vi "Table Select 2.vi"() -> ()   [LabVIEW 2019]
uses:
  Ctrl/Table Save.ctl
  LLB/Commonly VI.lvlib
panel:
  out "S14 Table":string[][](array[string])
  out "S1 Table":string[][](array[string])
  out "EnfMeasureTable":cluster{"Table Control":string[][]}[](array[cluster])
  in  "Tab Control":enum32{"Page 1", "Page 2", "Page 3", "Page 4"}(tab)
  out "S4 Table":string[][](array[string])
  out "S3 Table":string[][](array[string])
  out "S2 Table":string[][](array[string])
  out "S5 Table":string[][](array[string])
  out "S6 Table":string[][](array[string])
  out "S7 Table":string[][](array[string])
  out "S8 Table":string[][](array[string])
  out "S9 Table":string[][](array[string])
  out "S10 Table":string[][](array[string])
  out "S11 Table":string[][](array[string])
  out "S12 Table":string[][](array[string])
  out "S13 Table":string[][](array[string])
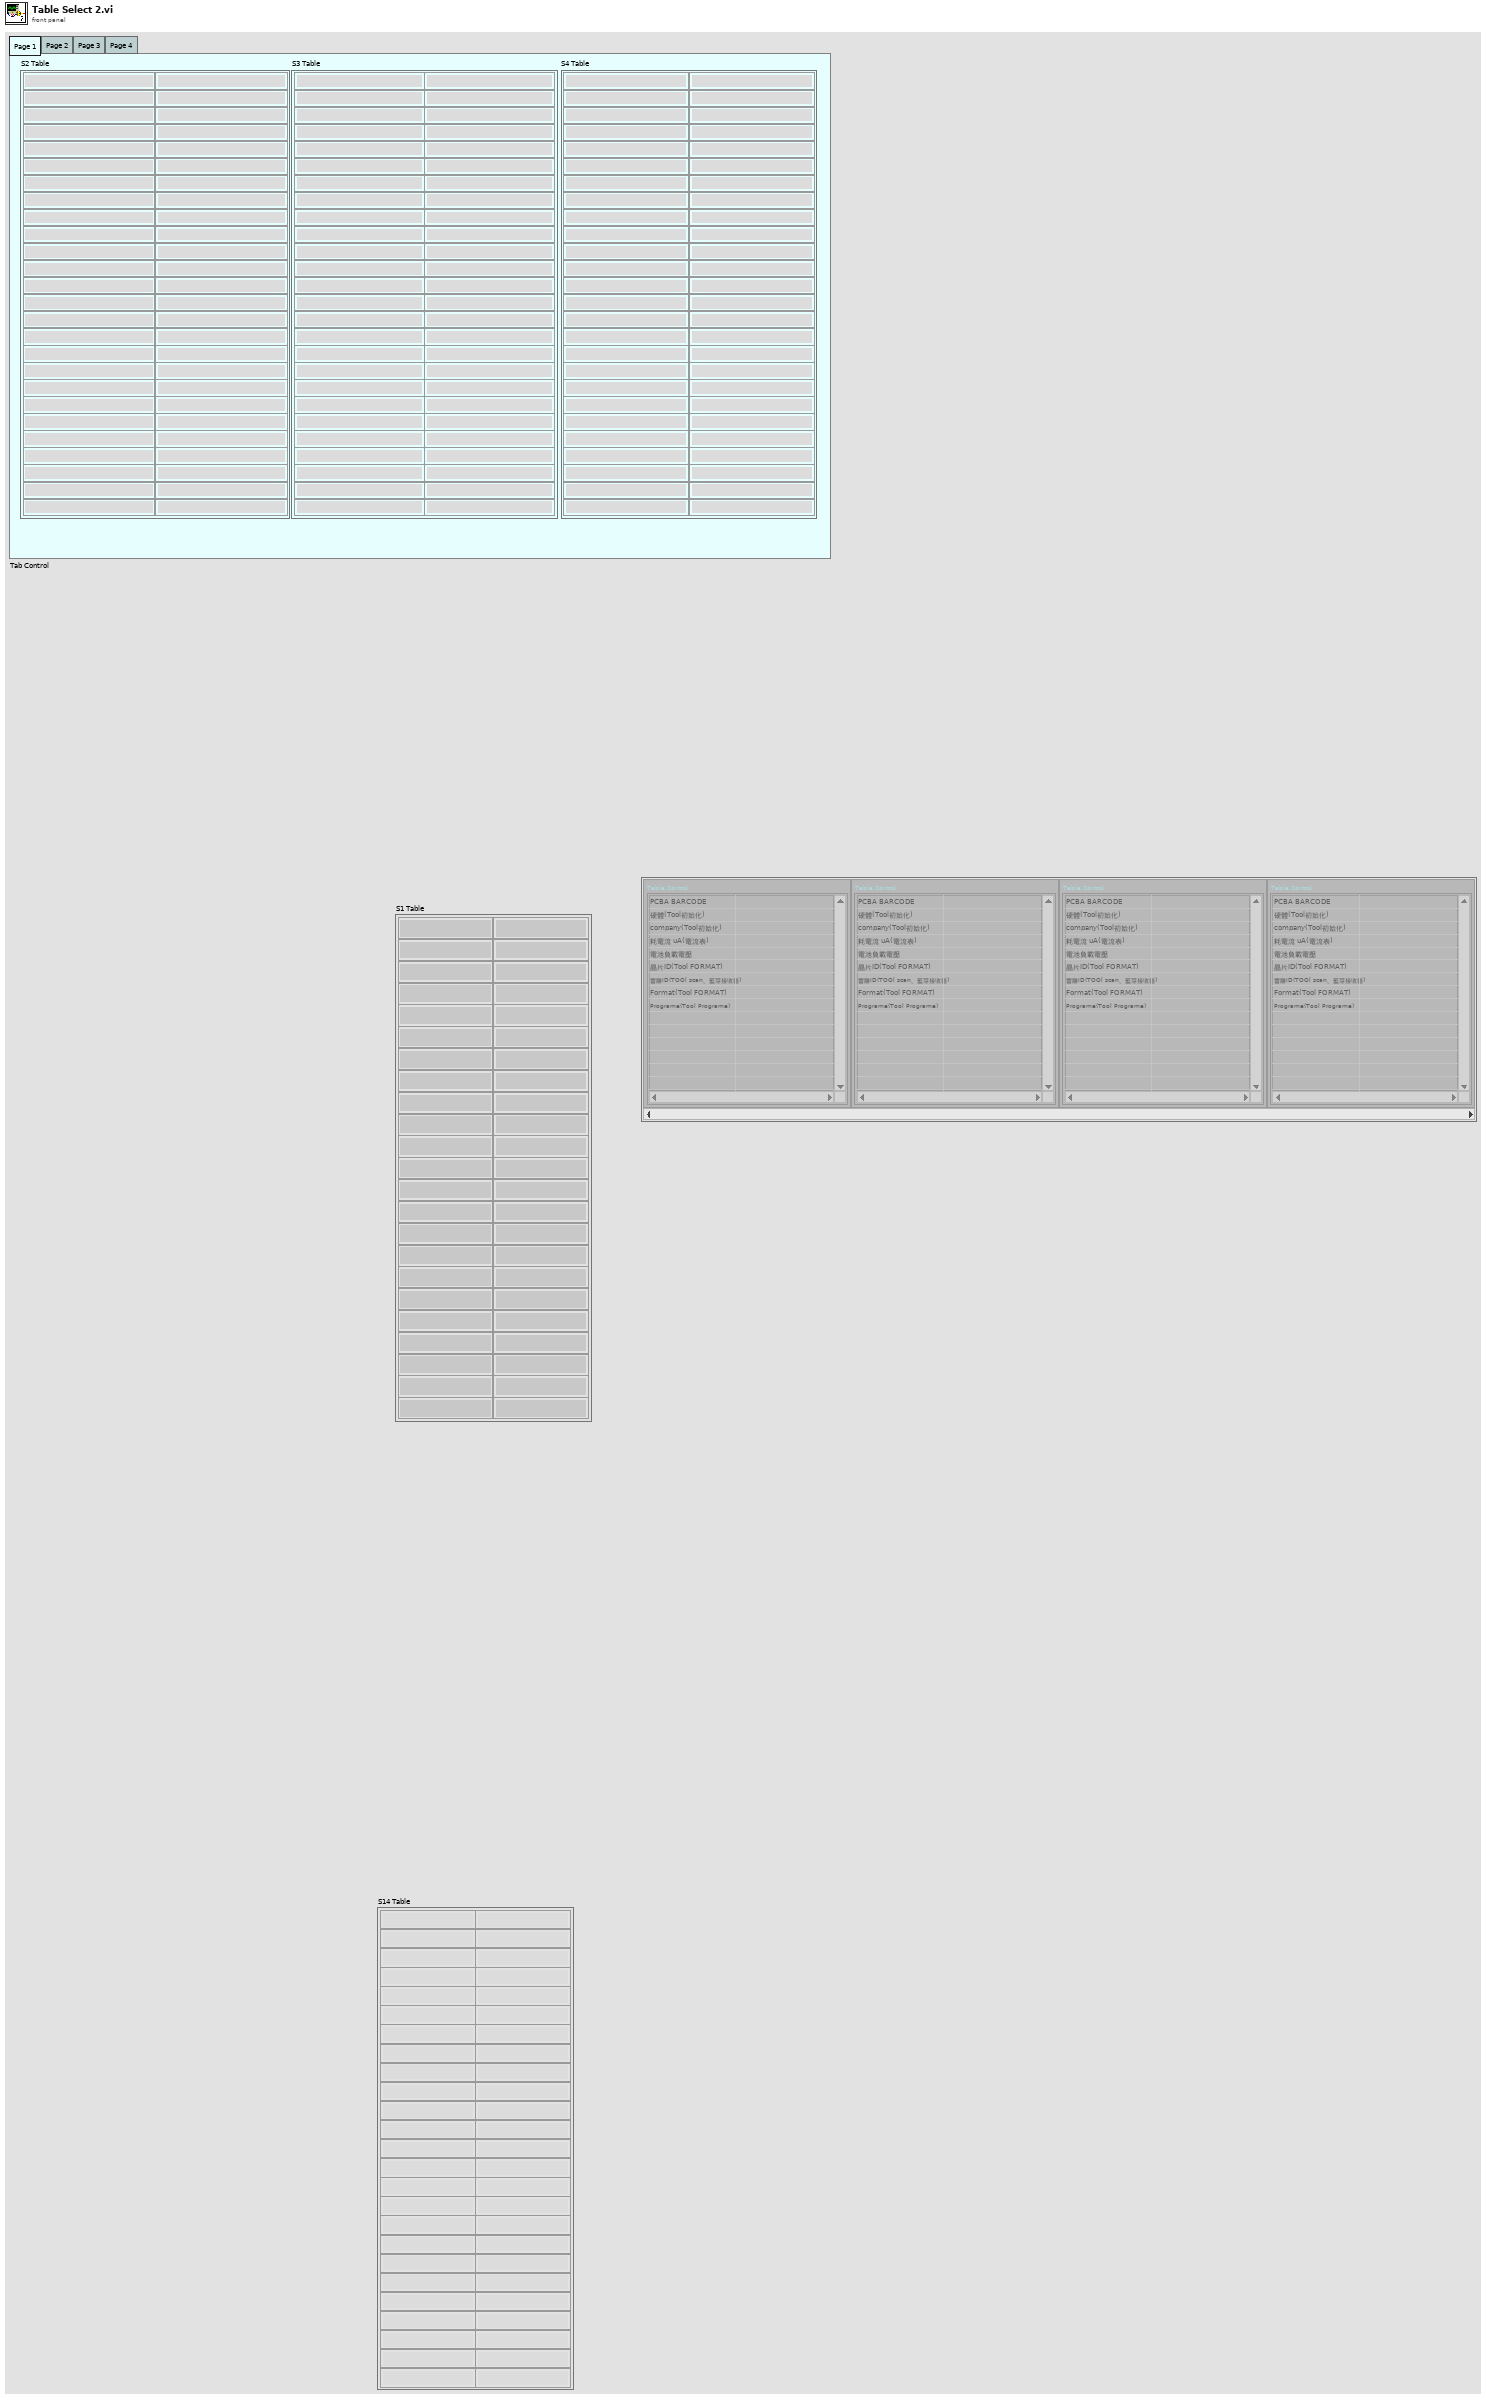
[diagram p1: front panel]
types:
  T1 = typedef "Table Save.ctl" = enum16{"initial", "Add", "Write", "Replace", "Delete", "REad", "RedTable", "Load"}
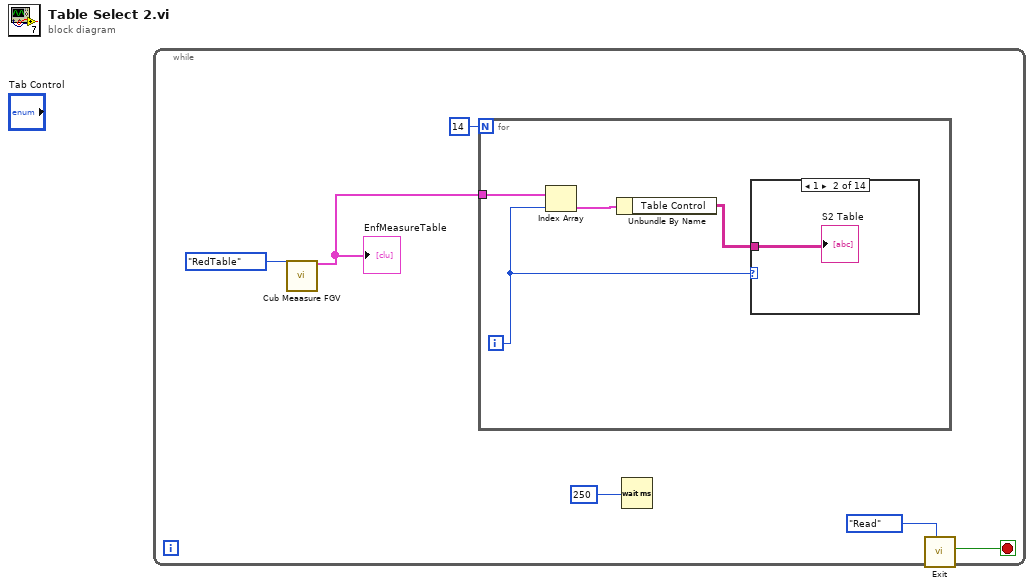
[diagram p0: block diagram]
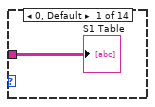
[diagram p2: hidden frame]
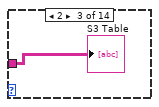
[diagram p3: hidden frame]
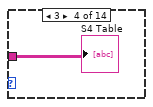
[diagram p4: hidden frame]
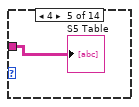
[diagram p5: hidden frame]
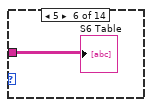
[diagram p6: hidden frame]
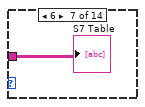
[diagram p7: hidden frame]
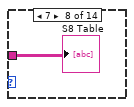
[diagram p8: hidden frame]
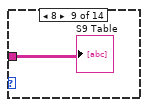
[diagram p9: hidden frame]
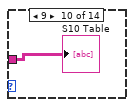
[diagram p10: hidden frame]
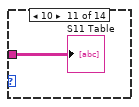
[diagram p11: hidden frame]
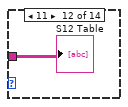
[diagram p12: hidden frame]
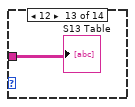
[diagram p13: hidden frame]
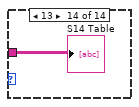
[diagram p14: hidden frame]
diagram:
  n1 = while {
    stop <- w2 stop-if-true
    n2 = call "Cub Meaasure FGV.vi"("Action"=Table_Save."RedTable" ("Enum")) -> ("Total Table"=w5:cluster{"Table Control":string[][]}[])  [unwired: 11 in, 7 out]
    "EnfMeasureTable" <- w5
    n3 = for {
      N: 14 -> [_]
      tunnel: w5 -> [w9]
      i -> [w8]
      n4 = Index Array(array=w9, index=w8) -> (element=w10:cluster{"Table Control":string[][]})
      n5 = Unbundle By Name(w10) -> ("Table Control"=w7:string[][])
      n6 = case shown="1" w8 {
        tunnel: w7 -> [w11 w12 w13 w14 w15 w16 w17 w18 w19 w20 w21 w22 w23 w24]
        frame 0, Default {
          "S1 Table" <- w11
        }
        frame 1 {
          "S2 Table" <- w12
        }
        frame 2 {
          "S3 Table" <- w13
        }
        frame 3 {
          "S4 Table" <- w14
        }
        frame 4 {
          "S5 Table" <- w15
        }
        frame 5 {
          "S6 Table" <- w16
        }
        frame 6 {
          "S7 Table" <- w17
        }
        frame 7 {
          "S8 Table" <- w18
        }
        frame 8 {
          "S9 Table" <- w19
        }
        frame 9 {
          "S10 Table" <- w20
        }
        frame 10 {
          "S11 Table" <- w21
        }
        frame 11 {
          "S12 Table" <- w22
        }
        frame 12 {
          "S13 Table" <- w23
        }
        frame 13 {
          "S14 Table" <- w24
        }
      }
    }
    n7 = Wait (ms)(milliseconds to wait=250) -> ()  [unwired: 1 out]
    n8 = call "Exit.vi"("Enum"=enum16{"Initial", "Read", "Write"}."Read") -> ("ExitOut"=w2:bool)  [unwired: 10 in]
  }
